vi "Find Path with Astar.vi"(8 "error in (no error)":errorcluster, 9 "goal node":cluster{"X":i32, "Y":i32}={"X"=32, "Y"=32}, 10 "start node":cluster{"X":i32, "Y":i32}={"X"=3, "Y"=3}, 11 "map reference in":refnum<data-value>) -> (0 "error out":errorcluster, 2 "intensity values":dbl[][](array[numeric]), 3 "map reference out":refnum<data-value>)   [LabVIEW 2016]
uses:
  <vilib>/robotics/Navigation/shared/WorldMap/OccupancyGridWorldMap/NI_Robotics_OccupancyGridWorldMap.lvclass
  C:/Program Files (x86)/National Instruments/LabVIEW 2016/vi.lib/robotics/Navigation/shared/WorldMap/AbstractWorldMap/NI_Robotics_AbstractWorldMap.lvclass
  <vilib>/robotics/Navigation/shared/MapNode/OccupancyGridNode/NI_Robotics_OccupancyGridMapNode.lvclass
  C:/Program Files (x86)/National Instruments/LabVIEW 2016/vi.lib/robotics/Navigation/shared/MapNode/AbstractAstarNode/NI_Robotics_AbstractAstarNode.lvclass
  <vilib>/robotics/Navigation/NI_Robotics_Navigation .lvlib
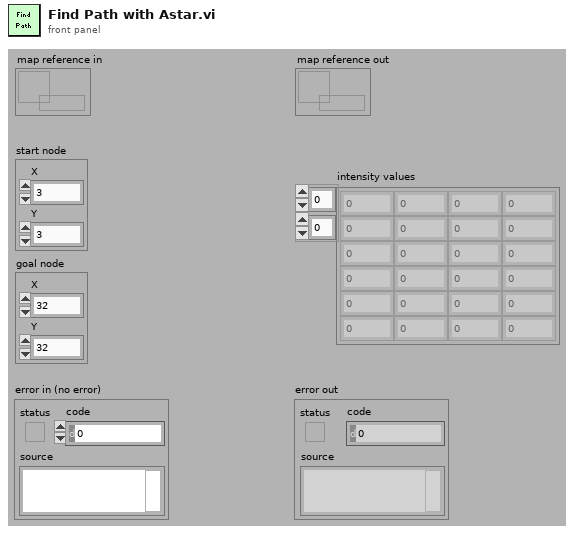
[diagram p1: front panel]
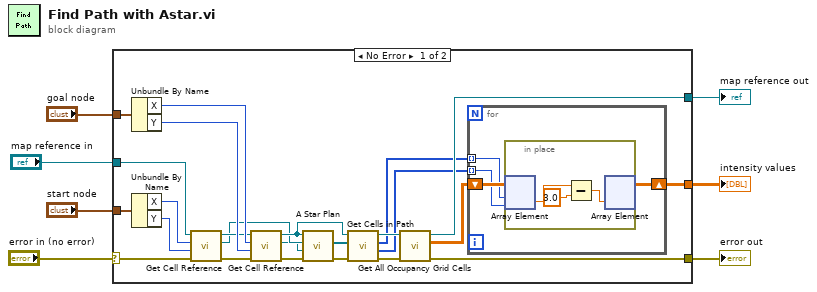
[diagram p0: block diagram]
diagram:
  n1 = case shown="No Error" "error in (no error)" {
    selector: "error in (no error)" -> [w15 w39]
    tunnel: "map reference in" -> [w16 w40]
    tunnel: "goal node" -> [w14 _]
    tunnel: "start node" -> [w13 _]
    tunnel: [w12 _] -> w3
    tunnel: [w11 w40] -> w2
    tunnel: [w10 w39] -> w1
    frame No Error {
      n2 = Unbundle By Name(w14) -> ("X"=w30:i32, "Y"=w31:i32)
      n3 = Unbundle By Name(w13) -> ("X"=w28:i32, "Y"=w29:i32)
      n4 = call <vilib>:"Get Cell Reference.vi"("error in (no error)"=w15, "y"=w29, "x"=w28, "map reference in"=w16) -> ("error out"=w20:errorcluster, "cell reference"=w18:refnum<data-value>, "map reference out"=w24:refnum<data-value>)  [unwired: 4 in, 1 out]
      n5 = call <vilib>:"Get Cell Reference.vi"("error in (no error)"=w20, "y"=w31, "x"=w30, "map reference in"=w24) -> ("error out"=w25:errorcluster, "cell reference"=w17:refnum<data-value>, "map reference out"=w22:refnum<data-value>)  [unwired: 4 in, 1 out]
      n6 = call <vilib>:"A Star Plan.vi"("error in (no error)"=w25, "goal reference"=w17, "start reference"=w18, "map reference in"=w22) -> ("error out"=w26:errorcluster, "path references"=w23:refnum<data-value>[])  [unwired: 4 in, 2 out]
      n7 = call <vilib>:"Get Cells in Path.vi"("error in (no error)"=w26, "path references"=w23, "map reference in"=w22) -> ("error out"=w19:errorcluster, "y coordinates"=w8:i32[], "x coordinates"=w9:i32[], "map reference out"=w21:refnum<data-value>)  [unwired: 5 in]
      n8 = call <vilib>:"Get All Occupancy Grid Cells.vi"("error in (no error)"=w19, "map reference in"=w21) -> ("error out"=w10:errorcluster, "occupancy grid"=w27:dbl[][], "map reference out"=w11:refnum<data-value>)  [unwired: 7 in]
      n9 = for {
        tunnel: w8 -> [w33] mode=indexing
        tunnel: w9 -> [w34] mode=indexing
        shift-right: [w32] -> w12
        shift-left: w27 -> [w35]
        n10 = in-place {
          n11 = in-place-array #1(w35, w34, w33) -> (w37:dbl)
          n12 = Subtract(x=w37, y=3.0) -> (x-y=w36:dbl)
          n13 = in-place-array #1(w36) -> (w32:dbl[][])  [unwired: 2 out]
        }
      }
    }
    frame Error {
    }
  }
  "error out" <- w1
  "intensity values" <- w3
  "map reference out" <- w2
